vi "image slider.vi"() -> ()   [LabVIEW 2022 SP3]
uses:
  <vilib>/picture/picture.llb/imagedata.ctl
panel:
  out "Gest":picture
  out "image data 2":T1
  out "String 2":string
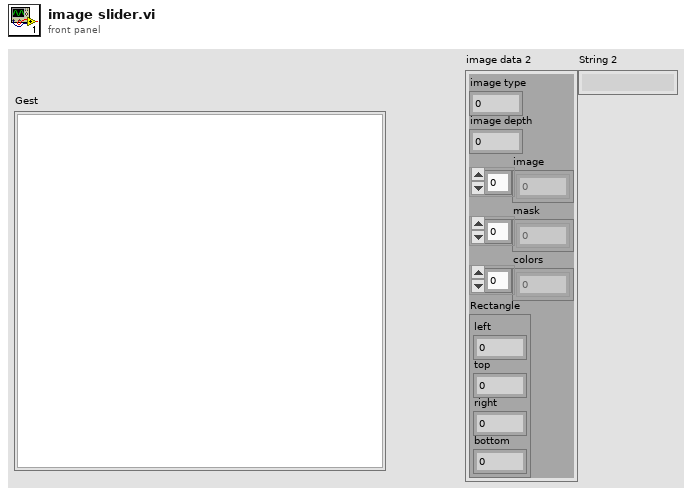
[diagram p1: front panel]
types:
  T1 = typedef "imagedata.ctl" = cluster{"image type":i32, "image depth":i32, "image":u8[], "mask":u8[], "colors":u32[], "Rectangle":cluster{"left":i16, "top":i16, "right":i16, "bottom":i16}}
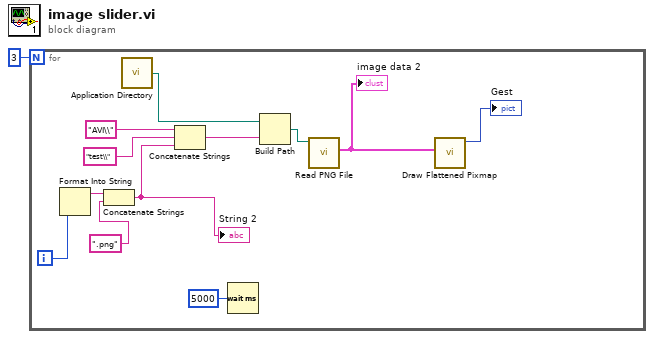
[diagram p0: block diagram]
diagram:
  n1 = for {
    N: 3 -> [_]
    i -> [w5]
    n2 = Format Into String(w5) -> (resulting string=w4:string)  [unwired: 3 in, 1 out]
    n3 = Concatenate Strings(w4, ".png" ("string")) -> (w2:string)
    "String 2" <- w2
    n4 = call <vilib>:"Application Directory.vi"() -> ("Application Directory"=w9:path)
    n5 = Concatenate Strings("AVI\\" ("string"), "test\\", w2) -> (w12:string)
    n6 = Wait (ms)(milliseconds to wait=u32 5000) -> ()  [unwired: 1 out]
    n7 = Build Path(base path=w9, name or relative path=w12) -> (appended path=w10:path)
    n8 = call <vilib>:"Read PNG File.vi"("path to PNG file"=w10) -> ("image data"=w13:T1)  [unwired: 8 in, 2 out]
    "image data 2" <- w13
    n9 = call <vilib>:"Draw Flattened Pixmap.vi"("image data"=w13) -> ("new picture"=→"Gest":picture)  [unwired: 8 in]
  }
